vi "Baidu_Map_GET.vi"() -> ()   [LabVIEW 2013]
uses:
  <vilib>/httpClient/LabVIEWHTTPClient.lvlib
panel:
  out "loops":i32
  in  "stop":bool
  out "error out":errorcluster
  out "hour":dbl
  out "minute":dbl
  out "toll_distance":string
  out "tollfee":string
  out "duration":string
  out "distance":string
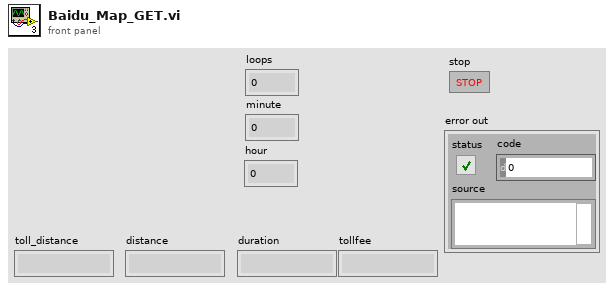
[diagram p1: front panel]
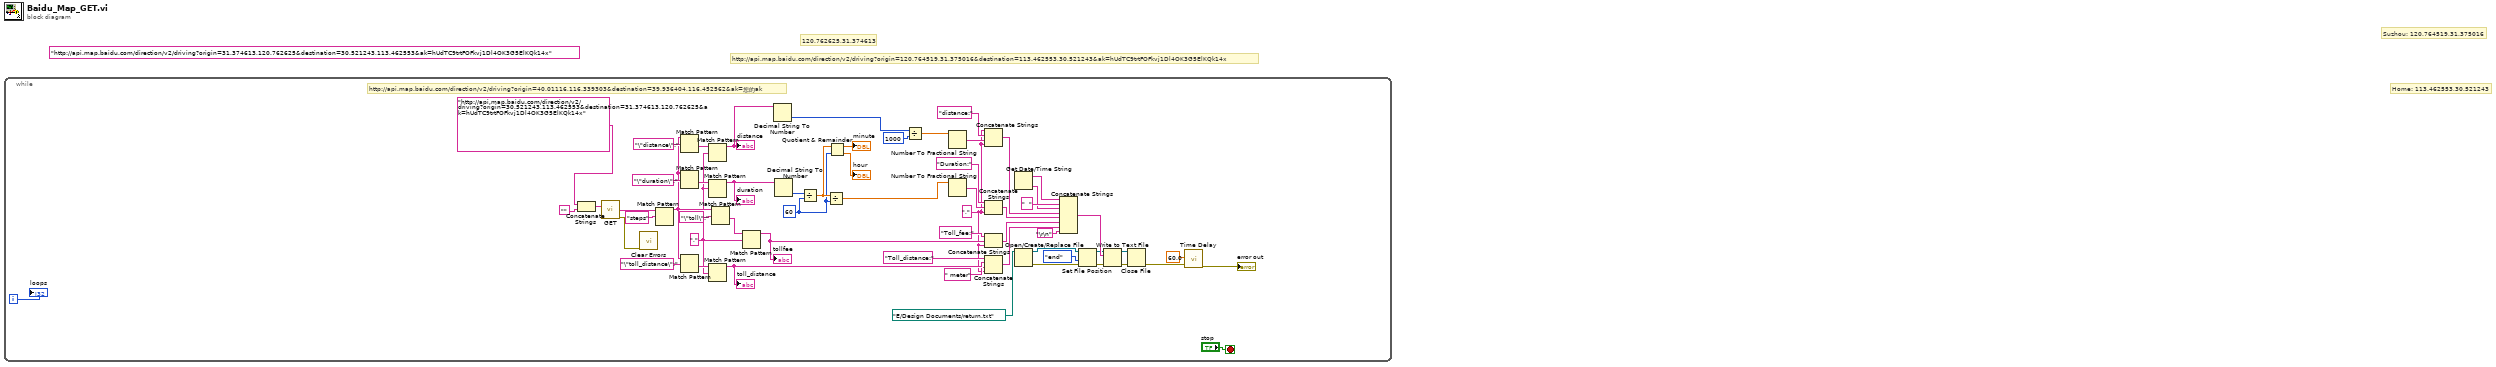
[diagram p0: block diagram]
diagram:
  (unwired) "http://api.map.baidu.com/direction/v2/driving?origin=31.374613,120.762625&destination=30.521243,113.462553&ak=hUdTC9trtFOFkvj1Dl4OK3G5ElKQk14x" ("string")
  # "120.762625,31.374613"
  # "http://api.map.baidu.com/direction/v2/driving?origin=40.01116,116.339303&destination=39.936404,116.452562&ak=您的ak"
  # "Home: 113.462553,30.521243"
  # "Suzhou: 120.764519,31.375016"
  # "http://api.map.baidu.com/direction/v2/driving?origin=120.764519,31.375016&destination=113.462553,30.521243&ak=hUdTC9trtFOFkvj1Dl4OK3G5ElKQk14x"
  n1 = while {
    i -> [w2]
    stop <- "stop" stop-if-true
    w21 = "," ("regular expression")
    w30 = 60 ("y")
    w46 = "," ("regular expression")
    n2 = Concatenate Strings("http://api.map.baidu.com/direction/v2/driving?origin=30.521243,113.462553&destination=31.374613,120.762625&ak=hUdTC9trtFOFkvj1Dl4OK3G5ElKQk14x" ("string"), "") -> (w59:string)
    n3 = call <vilib>:"GET.vi"("url"=w59) -> ("body"=w7:string, "error out"=w1:errorcluster)  [unwired: 11 in, 2 out]
    n4 = call <vilib>:"Clear Errors.vi"("error in (no error)"=w1) -> ()  [unwired: 6 in, 1 out]
    n5 = Match Pattern(string=w7, regular expression="steps") -> (before substring=w48:string)  [unwired: 1 in, 3 out]
    n6 = Match Pattern(string=w48, regular expression="\"distance\":") -> (after substring=w54:string)  [unwired: 1 in, 3 out]
    n7 = Match Pattern(string=w48, regular expression="\"duration\":") -> (after substring=w52:string)  [unwired: 1 in, 3 out]
    n8 = Match Pattern(string=w48, regular expression="\"toll_distance\":") -> (after substring=w47:string)  [unwired: 1 in, 3 out]
    n9 = Match Pattern(string=w54, regular expression=w46) -> (before substring=w38:string)  [unwired: 1 in, 3 out]
    "distance" <- w38
    n10 = Match Pattern(string=w52, regular expression=w46) -> (before substring=w45:string)  [unwired: 1 in, 3 out]
    "duration" <- w45
    n11 = Match Pattern(string=w47, regular expression=w46) -> (before substring=w23:string)  [unwired: 1 in, 3 out]
    "toll_distance" <- w23
    n12 = Match Pattern(string=w48, regular expression="\"toll\":") -> (after substring=w50:string)  [unwired: 1 in, 3 out]
    n13 = Match Pattern(string=w50, regular expression=w46) -> (before substring=w25:string)  [unwired: 1 in, 3 out]
    "tollfee" <- w25
    n14 = Decimal String To Number(string=w38) -> (number=w37:i32)  [unwired: 2 in, 1 out]
    n15 = Decimal String To Number(string=w45) -> (number=w44:i32)  [unwired: 2 in, 1 out]
    n16 = Divide(x=w44, y=w30) -> (x/y=w31:dbl)
    n17 = Divide(x=w31, y=w30) -> (x/y=w29:dbl)
    n18 = Quotient & Remainder(x=w31, y=w30) -> (x-y*floor(x/y)=→"minute":dbl, floor(x/y)=→"hour":dbl)
    n19 = Divide(x=w37, y=1000) -> (x/y=w35:dbl)
    n20 = Number To Fractional String(number=w35) -> (F-format string=w33:string)  [unwired: 3 in]
    n21 = Number To Fractional String(number=w29) -> (F-format string=w27:string)  [unwired: 3 in]
    n22 = Concatenate Strings(w21, "distance:" ("string"), w33, w21) -> (w32:string)
    n23 = Concatenate Strings("Duration:" ("string"), w27, w21) -> (w20:string)
    n24 = Concatenate Strings("Toll_fee:" ("string"), w25, w21) -> (w19:string)
    n25 = Concatenate Strings("Toll_distance:" ("string"), w23, " meter" ("string"), w21) -> (w18:string)
    n26 = Get Date/Time String() -> (date string=w41:string, time string=w39:string)  [unwired: 3 in]
    n27 = Open/Create/Replace File(file path (use dialog)=path "E:/Design Documents/return.txt") -> (refnum out=w14:refnum<file>, error out=w12:errorcluster)  [unwired: 5 in, 1 out]
    n28 = Concatenate Strings(w41, "  " ("string"), w39, w32, w20, w19, w18, "\r\n") -> (w15:string)
    n29 = Set File Position(refnum=w14, from (0:start)=enum16{"start", "end", "current"}."end", error in=w12) -> (refnum out=w13:refnum<file>, error out=w10:errorcluster)  [unwired: 1 in]
    n30 = Write to Text File(file (use dialog)=w13, text=w15, error in=w10) -> (refnum out=w9:refnum<file>, error out=w8:errorcluster)  [unwired: 1 in, 1 out]
    n31 = Close File(refnum=w9, error in=w8) -> (error out=w5:errorcluster)  [unwired: 1 out]
    n32 = call "Time Delay"("error in (no error)"=w5, "Delay Time (s)"=60.0) -> ("error out"=→"error out":errorcluster)  [unwired: 9 in]
    "loops" <- w2
  }
